vi "json Parse I64 Array - array path.vi"(8 "error in (no error)":errorcluster, 9 "default":i64[](array[numeric]), 10 "path":string[](array[string]), 11 "JSON Document in":refnum<class "JSON Document.lvclass">) -> (0 "error out":errorcluster, 1 "defaulted?":bool, 2 "value":i64[](array[numeric]), 3 "JSON Document out":refnum<class "JSON Document.lvclass">, 4 "elements defaulted?":bool[](array[boolean]))   [LabVIEW 2015, in "JSON Document.lvclass"]
uses:
  JSON Document.lvclass
  json Parse I64 Array - string path.vi
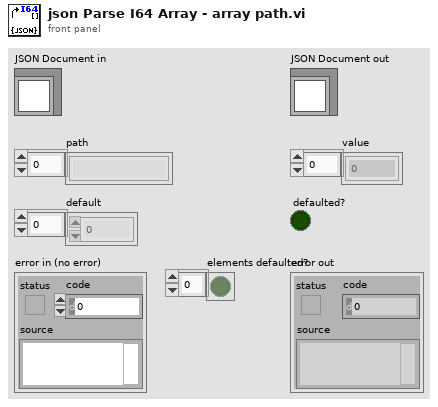
[diagram p1: front panel]
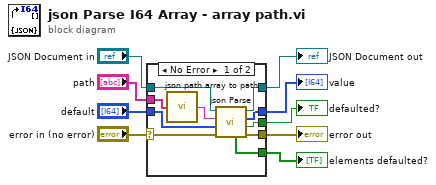
[diagram p0: block diagram]
diagram:
  n1 = case shown="No Error" "error in (no error)" {
    selector: "error in (no error)" -> [w10 w22]
    tunnel: [w11 w22] -> w8
    tunnel: [w15 w21] -> w6
    tunnel: "JSON Document in" -> [w16 w21]
    tunnel: "default" -> [w19 w20]
    tunnel: "path" -> [w18 _]
    tunnel: [w14 w20] -> w3
    tunnel: [w12 _] -> w2
    tunnel: [w13 _] -> w1
    frame No Error {
      n2 = call "json path array to path.vi"("path"=w18) -> ("String"=w17:string)
      n3 = call-poly "json Parse.vi"("error in (no error)"=w10, "default"=w19, "path"=w17, "JSON Document in"=w16) -> ("error out"=w11:errorcluster, "defaulted?"=w12:bool, "value"=w14:i64[], "JSON Document out"=w15:refnum<class "JSON Document.lvclass">, "elements defaulted?"=w13:bool[])  [unwired: 3 in]
    }
    frame Error {
    }
  }
  "error out" <- w8
  "JSON Document out" <- w6
  "value" <- w3
  "defaulted?" <- w2
  "elements defaulted?" <- w1
